vi "t.vi"() -> ()   [LabVIEW 2012]
panel:
  in  "Arean":dbl
  in  "Pin":dbl
  out "Verkningsgrad":dbl
  out "FF":dbl
  in  "Spänningintervall":dbl(slide) scale=0.0..10.0
  in  "Boolean":bool
  in  "Antal mätpunkter":dbl
  in  "R":dbl(slide) scale=0.0..10.0
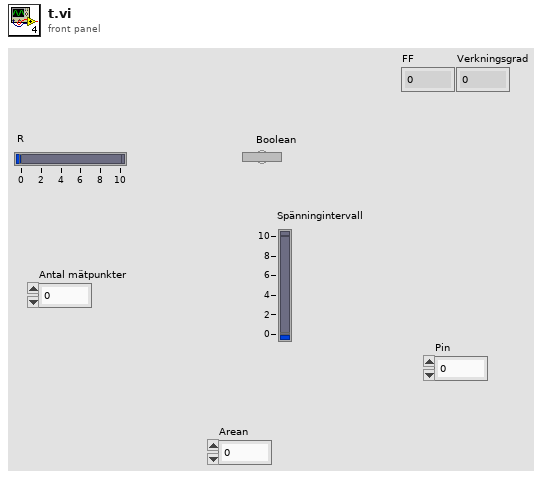
[diagram p1: front panel]
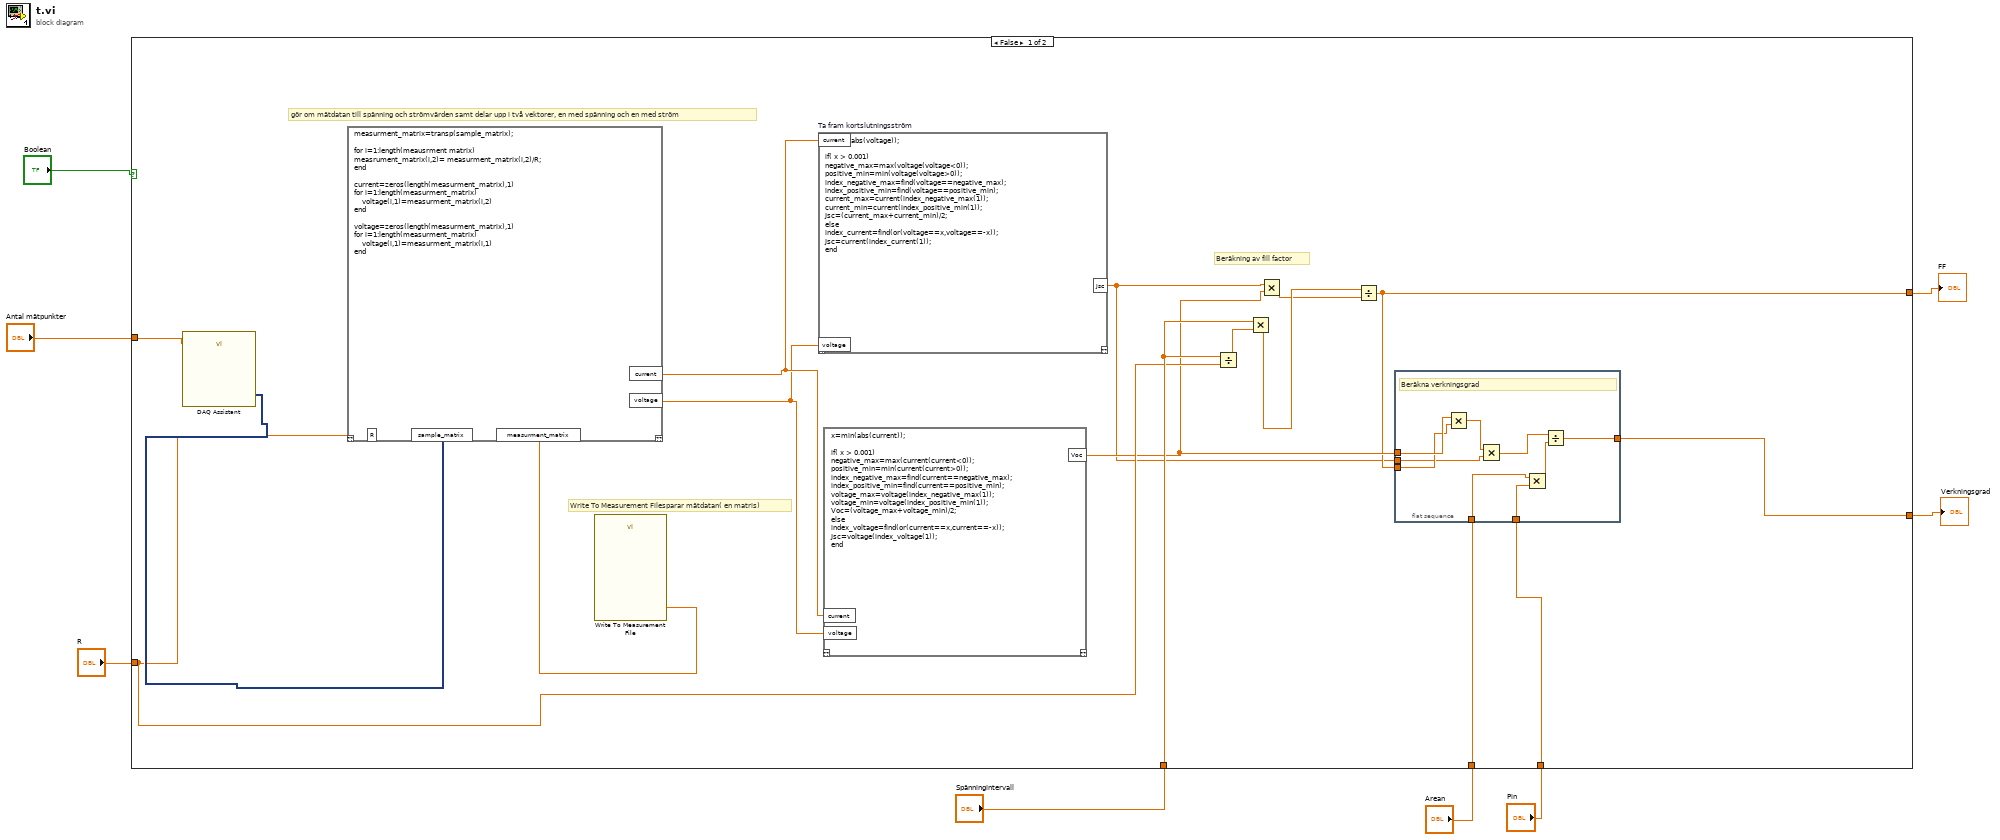
[diagram p0: block diagram]
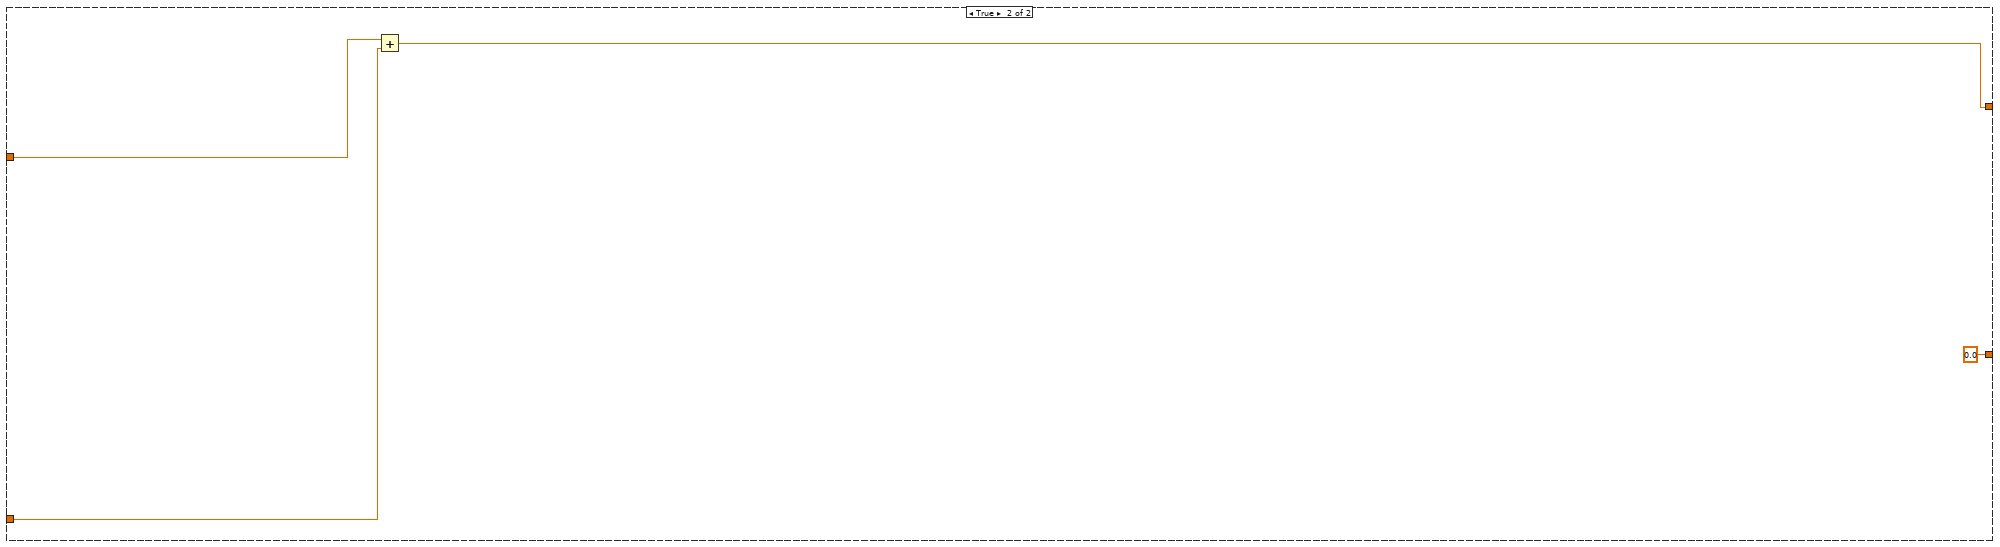
[diagram p2: hidden frame]
diagram:
  n1 = case shown="False" "Boolean" {
    tunnel: [w24 0.0] -> w3
    tunnel: "R" -> [w17 w36]
    tunnel: "Antal mätpunkter" -> [w22 w37]
    tunnel: "Spänningintervall" -> [w18 _]
    tunnel: [w14 w35] -> w4
    tunnel: "Pin" -> [w12 _]
    tunnel: "Arean" -> [w11 _]
    frame False {
      # "Beräkning av fill factor"
      # "Write To Measurement Filesparar mätdatan( en matris)"
      # "gör om mätdatan till spänning och strömvärden samt delar upp i två vektorer, en med spänning och en med ström"
      n2 = call "DAQ Assistant"("number of samples"=w22) -> ("data"=w23:dynamicdata)  [unwired: 16 in, 2 out]
      n3 = script code="measurment_matrix=transp(sample_matrix);\n\nfor i=1:length(meausrment matrix)\nmeasrument_matrix(i,2)= measurment_matrix(i,2)/R;\nend \n\ncurrent=zeros(length(measurment_matrix),1)\nfor i=1:length(measurment_matrix)\n    voltage(i,1)=measurment_matrix(i,2)\nend\n\nvoltage=zeros(length(measurment_matrix),1)\nfor i=1:length(measurment_matrix)\n    voltage(i,1)=measurment_matrix(i,1)\nend"("sample_matrix"=w23, "R"=w17) -> ("measurment_matrix"=w21:dbl, "current"=w10:dbl, "voltage"=w9:dbl)  [unwired: 1 in, 1 out]
      n4 = call "Write To Measurement File"("Signals"=w21) -> ()  [unwired: 16 in, 3 out]
      n5 = script code="x=min(abs(voltage));\n\nif( x > 0.001)\nnegative_max=max(voltage(voltage<0));\npositive_min=min(voltage(voltage>0));\nindex_negative_max=find(voltage==negative_max);\nindex_positive_min=find(voltage==positive_min);\ncurrent_max=current(index_negative_max(1));\ncurrent_min=current(index_positive_min(1));\nJsc=(current_max+current_min)/2;\nelse\nindex_current=find(or(voltage==x,voltage==-x));\nJsc=current(index_current(1));\nend" "Ta fram kortslutningsström"("current"=w10, "voltage"=w9) -> ("Jsc"=w13:dbl)  [unwired: 1 in, 1 out]
      n6 = script code="x=min(abs(current));\n\nif( x > 0.001)\nnegative_max=max(current(current<0));\npositive_min=min(current(current>0));\nindex_negative_max=find(current==negative_max);\nindex_positive_min=find(current==positive_min);\nvoltage_max=voltage(index_negative_max(1));\nvoltage_min=voltage(index_positive_min(1));\nVoc=(voltage_max+voltage_min)/2;\nelse\nindex_voltage=find(or(current==x,current==-x));\nJsc=voltage(index_voltage(1));\nend"("current"=w10, "voltage"=w9) -> ("Voc"=w15:dbl)  [unwired: 1 in, 1 out]
      n7 = Divide(x=w18, y=w17) -> (x/y=w16:dbl)
      n8 = Multiply(x=w18, y=w16) -> (x*y=w20:dbl)
      n9 = Multiply(x=w13, y=w15) -> (x*y=w19:dbl)
      n10 = Divide(x=w20, y=w19) -> (x/y=w14:dbl)
      n11 = flat-sequence {
        tunnel: [w31] -> w24
        tunnel: w15 -> [w29]
        tunnel: w14 -> [w28]
        tunnel: w13 -> [w27]
        tunnel: w12 -> [w26]
        tunnel: w11 -> [w25]
        frame #0 {
          # "Beräkna verkningsgrad"
          n12 = Multiply(x=w29, y=w28) -> (x*y=w33:dbl)
          n13 = Multiply(x=w33, y=w27) -> (x*y=w32:dbl)
          n14 = Multiply(x=w25, y=w26) -> (x*y=w30:dbl)
          n15 = Divide(x=w32, y=w30) -> (x/y=w31:dbl)
        }
      }
    }
    frame True {
      n16 = Add(x=w37, y=w36) -> (x+y=w35:dbl)
    }
  }
  "FF" <- w4
  "Verkningsgrad" <- w3
